vi "_PluginLoader_GetPluginsForType.vi"(8 "error in (no error)":errorcluster, 10 "ProjectItem":refnum<vi>, 11 "_PluginLoader in":refnum<class "_PluginLoader.lvclass">) -> (0 "error out":errorcluster, 1 "Plugins":refnum<class "GCMPlugin.lvclass">[](array[class]), 2 "ProjectItem out":refnum<vi>, 3 "_PluginLoader out":refnum<class "_PluginLoader.lvclass">)   [LabVIEW 2014, in "_PluginLoader.lvclass"]
uses:
  _PluginLoader.lvclass
  GCMPlugin/GCMPlugin.lvclass
  _PluginLoader.lvclass/_PluginLoader.ctl
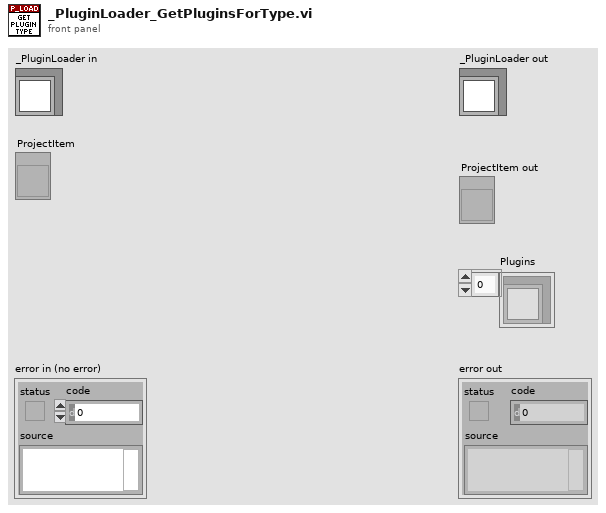
[diagram p1: front panel]
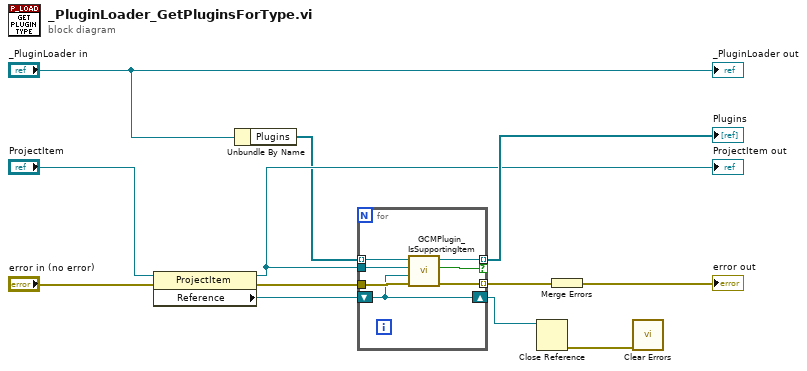
[diagram p0: block diagram]
diagram:
  n1 = property class="ProjectItem"(reference="ProjectItem", error in="error in (no error)") -> (reference out=w7:refnum<vi>, error out=w4:errorcluster, "Reference"=w3:refnum<vi>)
  "ProjectItem out" <- w7
  n2 = Unbundle By Name("_PluginLoader in") -> ("Plugins"=w6:refnum<class "GCMPlugin.lvclass">[])
  n3 = for {
    tunnel: w6 -> [w19] mode=indexing
    tunnel: [w15] -> w10 mode=indexing if=w14
    tunnel: w4 -> [w18]
    tunnel: [w16] -> w5 mode=indexing
    tunnel: w7 -> [w13]
    shift-right: [w17] -> w2
    shift-left: w3 -> [w17]
    n4 = call-dynamic "GCMPlugin_IsSupportingItem.vi"("error in (no error)"=w18, "VI Reference"=w17, "ProjectItem Refnum"=w13, "_LVCMPlugin in"=w19) -> ("error out"=w16:errorcluster, "IsSupportingItem"=w14:bool, "_LVCMPlugin out"=w15:refnum<class "GCMPlugin.lvclass">)  [unwired: 5 in]
  }
  "Plugins" <- w10
  n5 = Close Reference(reference=w2) -> (error out=w1:errorcluster)  [unwired: 1 in]
  n6 = Merge Errors(w5) -> (→"error out":errorcluster)
  n7 = call <vilib>:"Clear Errors.vi"("error in (no error)"=w1) -> ()  [unwired: 5 in, 2 out]
  "_PluginLoader out" <- "_PluginLoader in"
